vi "Read.vi"(8 "error in (no error)":errorcluster, 11 "Waveform Array in":refnum<class "Waveform Array.lvclass">) -> (0 "error out":errorcluster, 2 "Waveform Array":waveform(dbl)[](array[waveform]), 3 "Waveform Array out":refnum<class "Waveform Array.lvclass">)   [LabVIEW 2020, in "Data.lvlib" / "Waveform Array.lvclass"]
doc: "Read Waveform Array."
uses:
  Waveform Array.lvclass
  Waveform Array.lvclass/Waveform Array.ctl
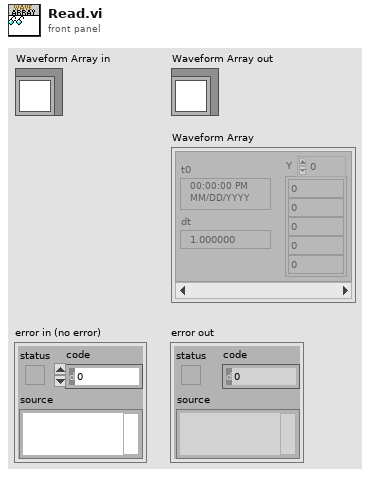
[diagram p1: front panel]
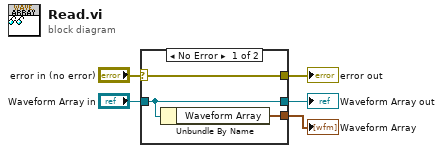
[diagram p0: block diagram]
diagram:
  n1 = case shown="No Error" "error in (no error)" {
    selector: "error in (no error)" -> [w8 w9]
    tunnel: [w8 w9] -> w4
    tunnel: [w7 w10] -> w2
    tunnel: "Waveform Array in" -> [w7 w10]
    tunnel: [w6 _] -> w1
    frame No Error {
      n2 = Unbundle By Name(w7) -> ("Waveform Array"=w6:waveform(dbl)[])
    }
    frame Error {
    }
  }
  "error out" <- w4
  "Waveform Array out" <- w2
  "Waveform Array" <- w1
